vi "PKG_IMC_GetLogicVel.vi"(9 "axisnum":i32, 10 "vel":dbl[](array[numeric])=array[4097 elements], 11 "Handle":u32) -> (1 "function return":i32, 2 "vel out":dbl[](array[numeric]), 3 "Handle out":u32)   [LabVIEW 2011, in "IMC_Pkg4xxx.lvlib"]
doc: "PKG_IMC_GetLogicVel(IMC_HANDLE Handle, double vel[], int axisnum);"
uses:
  IMC_Pkg4xxx.lvlib
  IMC_Pkg4xxx.dll
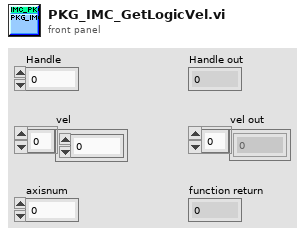
[diagram p1: front panel]
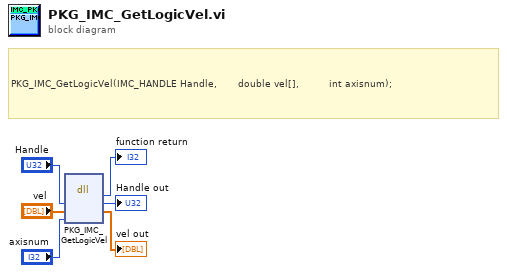
[diagram p0: block diagram]
diagram:
  # "PKG_IMC_GetLogicVel(IMC_HANDLE Handle,  \t\t\t\t\tdouble vel[],  \t\t\t\t\t\t\t\tint axisnum);"
  n1 = dll-call lib="PTH1mabs F光盘刻录\niMC MotionIMCNet_V4.0IMCAppincLabviewIMC_PKG4xxxIMC_PKG4xxx\nIMC_Pkg4xxx.*" fn="PKG_IMC_GetLogicVel"("Handle"="Handle", "vel"="vel", "axisnum"="axisnum") -> (→"function return":i32, "Handle"=→"Handle out":u32, "vel"=→"vel out":dbl[])  [unwired: 4 in, 2 out]
